vi "Fs_to_FilterDelay.vi"(8 "error in (no error)":errorcluster, 10 "Fs":dbl, 11 "Refnum in":refnum<k21>) -> (0 "error out":errorcluster, 2 "Total Filter Delay (samples)":i32, 3 "Refnum out":refnum<k21>)   [LabVIEW 2019, in "Instrument.DAQ.lvclass"]
uses:
  Instrument.DAQ.lvclass
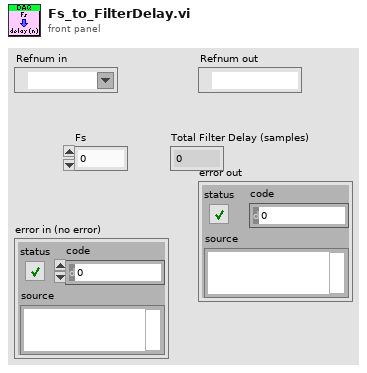
[diagram p1: front panel]
types:
  T1 = typedef "Instrument.DAQ.lvclass/DAQ.Type--enum.ctl" = enum16{"None", "USB 4431", "PXI 446x"}
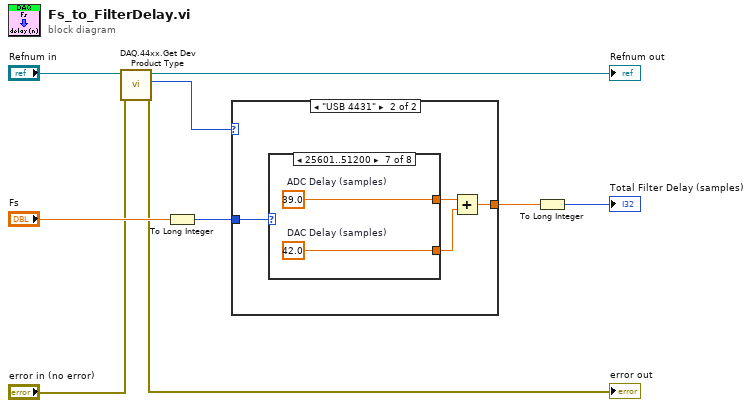
[diagram p0: block diagram]
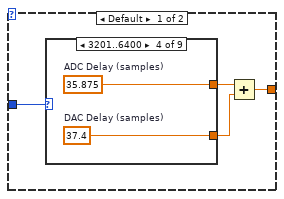
[diagram p2: hidden frame]
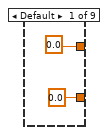
[diagram p3: hidden frame]
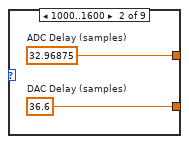
[diagram p4: hidden frame]
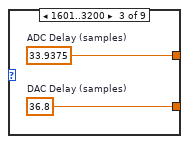
[diagram p5: hidden frame]
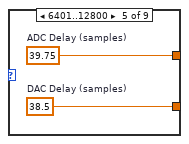
[diagram p6: hidden frame]
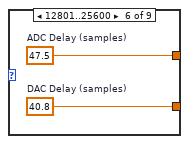
[diagram p7: hidden frame]
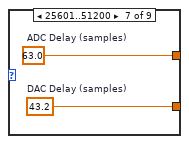
[diagram p8: hidden frame]
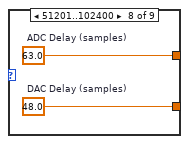
[diagram p9: hidden frame]
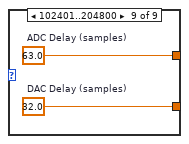
[diagram p10: hidden frame]
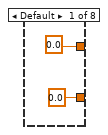
[diagram p11: hidden frame]
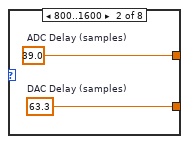
[diagram p12: hidden frame]
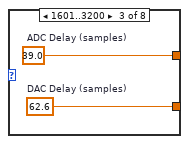
[diagram p13: hidden frame]
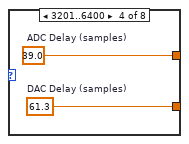
[diagram p14: hidden frame]
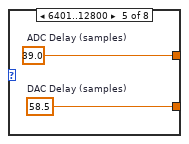
[diagram p15: hidden frame]
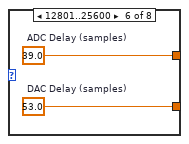
[diagram p16: hidden frame]
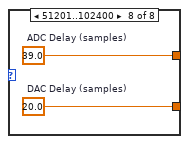
[diagram p17: hidden frame]
diagram:
  n1 = call "DAQ.44xx.Get Dev Product Type.vi"("error in (no error)"="error in (no error)", "Refnum in"="Refnum in") -> ("error out"=→"error out":errorcluster, "DAQ Type"=w7:T1, "Refnum out"=→"Refnum out":refnum<k21>)  [unwired: 6 in, 1 out]
  n2 = To Long Integer(number="Fs") -> (32bit integer=w8:i32)
  n3 = case shown="\"USB 4431\"" w7 {
    tunnel: w8 -> [w11 w33]
    tunnel: [w10 w32] -> w2
    frame Default {
      n4 = case shown="3201..6400" w11 {
        tunnel: [0.0 ("ADC Delay (samples)") w17 w19 w21 w23 w25 w27 w29 w31] -> w12
        tunnel: [0.0 ("ADC Delay (samples)") w16 w18 w20 w22 w24 w26 w28 w30] -> w13
        frame Default {
        }
        frame 1000..1600 {
          w16 = 36.6  # DAC Delay (samples)
          w17 = 32.96875  # ADC Delay (samples)
        }
        frame 1601..3200 {
          w18 = 36.8  # DAC Delay (samples)
          w19 = 33.9375  # ADC Delay (samples)
        }
        frame 3201..6400 {
          w20 = 37.4  # DAC Delay (samples)
          w21 = 35.875  # ADC Delay (samples)
        }
        frame 6401..12800 {
          w22 = 38.5  # DAC Delay (samples)
          w23 = 39.75  # ADC Delay (samples)
        }
        frame 12801..25600 {
          w24 = 40.8  # DAC Delay (samples)
          w25 = 47.5  # ADC Delay (samples)
        }
        frame 25601..51200 {
          w27 = 63.0  # ADC Delay (samples)
          w26 = 43.2  # DAC Delay (samples)
        }
        frame 51201..102400 {
          w29 = 63.0  # ADC Delay (samples)
          w28 = 48.0  # DAC Delay (samples)
        }
        frame 102401..204800 {
          w31 = 63.0  # ADC Delay (samples)
          w30 = 32.0  # DAC Delay (samples)
        }
      }
      n5 = Add(x=w12, y=w13) -> (x+y=w10:dbl)
    }
    frame "USB 4431" {
      n6 = case shown="25601..51200" w33 {
        tunnel: [0.0 ("ADC Delay (samples)") w39 w41 w43 w45 w47 w49 w51] -> w34
        tunnel: [0.0 ("ADC Delay (samples)") w38 w40 w42 w44 w46 w48 w50] -> w35
        frame Default {
        }
        frame 800..1600 {
          w38 = 63.3  # DAC Delay (samples)
          w39 = 39.0  # ADC Delay (samples)
        }
        frame 1601..3200 {
          w40 = 62.6  # DAC Delay (samples)
          w41 = 39.0  # ADC Delay (samples)
        }
        frame 3201..6400 {
          w42 = 61.3  # DAC Delay (samples)
          w43 = 39.0  # ADC Delay (samples)
        }
        frame 6401..12800 {
          w44 = 58.5  # DAC Delay (samples)
          w45 = 39.0  # ADC Delay (samples)
        }
        frame 12801..25600 {
          w46 = 53.0  # DAC Delay (samples)
          w47 = 39.0  # ADC Delay (samples)
        }
        frame 25601..51200 {
          w49 = 39.0  # ADC Delay (samples)
          w48 = 42.0  # DAC Delay (samples)
        }
        frame 51201..102400 {
          w51 = 39.0  # ADC Delay (samples)
          w50 = 20.0  # DAC Delay (samples)
        }
      }
      n7 = Add(x=w34, y=w35) -> (x+y=w32:dbl)
    }
  }
  n8 = To Long Integer(number=w2) -> (32bit integer=→"Total Filter Delay (samples)":i32)
